vi "Dialog_Enter Wait Duration.vi"(8 "Error In":errorcluster) -> (0 "Error Out":errorcluster, 2 "Cancelled?":bool, 3 "Macro Commands":T1)   [LabVIEW 2012]
doc: "This VI has no controls.\nThis is a dummy whihc runs when user selects a macro command which does not require any arguments"
uses:
  Custom Controls and Typedefs/Macro_CommandStruct.ctl
  Custom Controls and Typedefs/Macro_Action_List.ctl
  Custom Controls and Typedefs/Macro_ArgumentStruct.ctl
panel:
  in  "Cancel Button":bool
  in  "OK Button":bool
  in  "Seconds to Wait":dbl
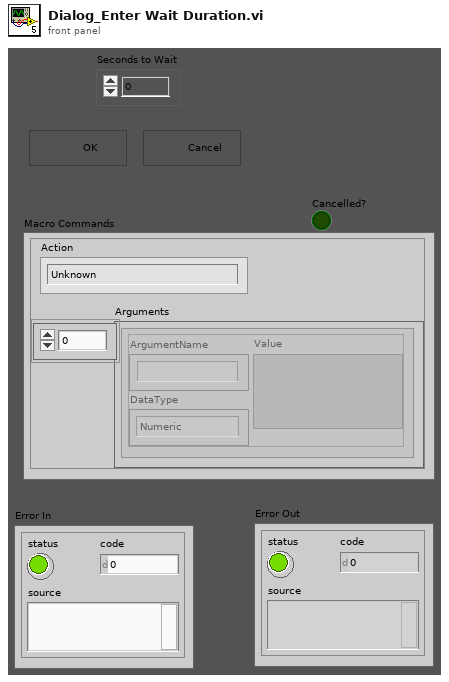
[diagram p1: front panel]
types:
  T1 = typedef "Macro_CommandStruct.ctl" = cluster{"Action":T2, "Arguments":T3[]}
  T2 = typedef "Macro_Action_List.ctl" = enum16{"Unknown", "2D.Frame.Scan", "2D.Line.Scan", "Load.Settings.File", "Move.To.Position", "Pause", "Z.Stack", "LOOP.Start", "LOOP.End"}
  T3 = typedef "Macro_ArgumentStruct.ctl" = cluster{"ArgumentName":string, "DataType":enum16{"Numeric", "String"}, "Value":variant}
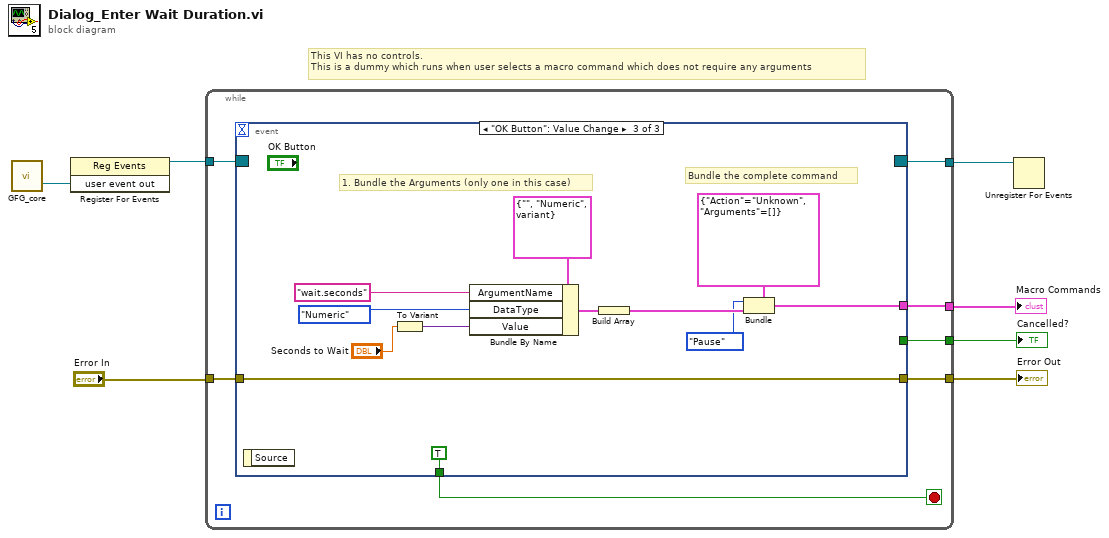
[diagram p0: block diagram]
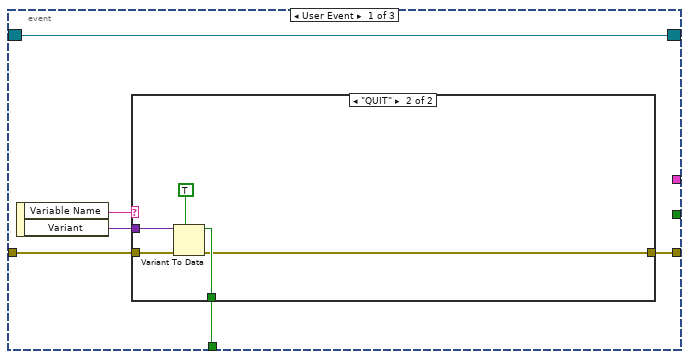
[diagram p2: hidden frame]
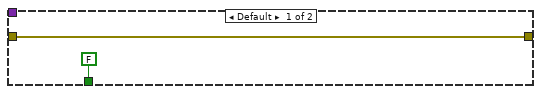
[diagram p3: hidden frame]
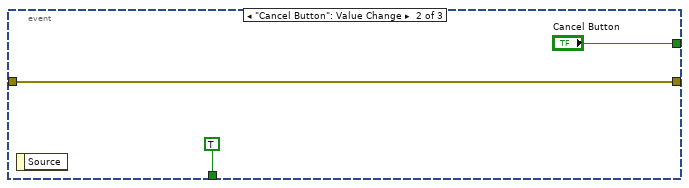
[diagram p4: hidden frame]
diagram:
  # "This VI has no controls.\nThis is a dummy which runs when user selects a macro command which does not require any arguments"
  n1 = call "GFG_core.vi"() -> ("user event out"=w7:refnum<user-event>)  [unwired: 13 in, 6 out]
  n2 = register-events(w7) -> (reference out=w6:refnum<event-registration>)  [unwired: 2 in, 1 out]
  n3 = while {
    tunnel: w6 -> [w14]
    tunnel: [w13] -> w5
    tunnel: "Error In" -> [w11]
    tunnel: [w10] -> w3
    tunnel: [w9] -> w2
    tunnel: [w8] -> w1
    stop <- w12 stop-if-true
    n4 = event shown="[2] \"OK Button\": Value Change" {
      selector: w14 -> [w20 _ _]
      dyn-events: [w20 _ _] -> w13
      timeout: _ -> [_ _ _]
      tunnel: [w17 TRUE TRUE] -> w12
      tunnel: w11 -> [w16 w29 w32]
      tunnel: [w15 w29 w32] -> w10
      tunnel: [_ _ w33] -> w9
      tunnel: [_ "Cancel Button" _] -> w8
      event User Event {
        n5 = event-data() -> ("Variable Name"=w19:string, "Variant"=w18:variant)  [unwired: 1 in]
        n6 = case shown="\"QUIT\"" w19 {
          tunnel: w18 -> [_ w26]
          tunnel: [FALSE w25] -> w17
          tunnel: w16 -> [w21 w24]
          tunnel: [w21 w23] -> w15
          frame Default {
          }
          frame "QUIT" {
            n7 = Variant To Data(error in=w24, type=TRUE, Variant=w26) -> (data=w25:bool, error out=w23:errorcluster)
          }
        }
      }
      event "Cancel Button": Value Change {
        n8 = event-data() -> ()  [unwired: 1 in, 1 out]
      }
      event "OK Button": Value Change {
        # "Bundle the complete command"
        # "1. Bundle the Arguments (only one in this case)"
        n9 = event-data() -> ()  [unwired: 1 in, 1 out]
        n10 = To Variant(anything="Seconds to Wait") -> (Variant=w38:variant)
        n11 = Bundle By Name(cluster=T3 {"ArgumentName"="", "DataType"=enum."Numeric", "Value"=variant} ("Arguments"), "ArgumentName"="wait.seconds", "DataType"=enum16{"Numeric", "String"}."Numeric", "Value"=w38) -> (w36:T3)
        n12 = Build Array(w36) -> (w35:T3[])
        n13 = Bundle(cluster=T1 {"Action"=enum."Unknown", "Arguments"=[]} ("Macro Commands"), "Action"=Macro_Action_List."Pause", "Arguments"=w35) -> (w33:T1)
      }
    }
  }
  "Error Out" <- w3
  "Macro Commands" <- w2
  "Cancelled?" <- w1
  n14 = Unregister For Events(event registration refnum=w5) -> ()  [unwired: 1 in, 1 out]
